vi "setWindow.vi"(8 "error in (no error)":errorcluster, 10 "Window Number (0...15)":i32, 11 "Stimulus in":refnum<class "Stimulus.lvclass">) -> (0 "error out":errorcluster, 3 "Stimulus out":refnum<class "Stimulus.lvclass">)   [LabVIEW 2013, in "Stimulus.lvclass"]
uses:
  Stimulus.lvclass
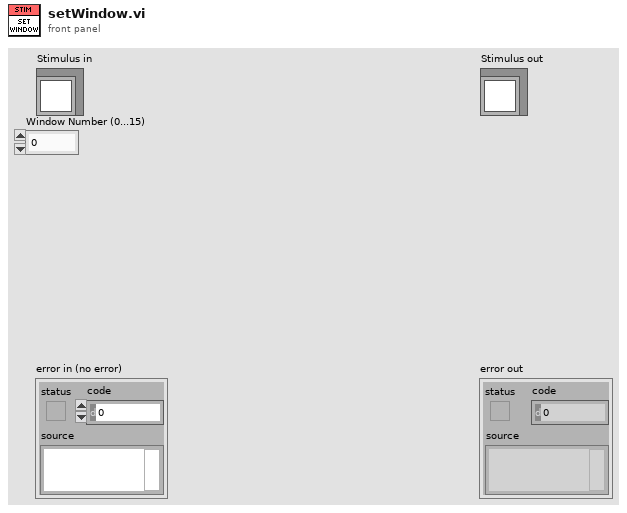
[diagram p1: front panel]
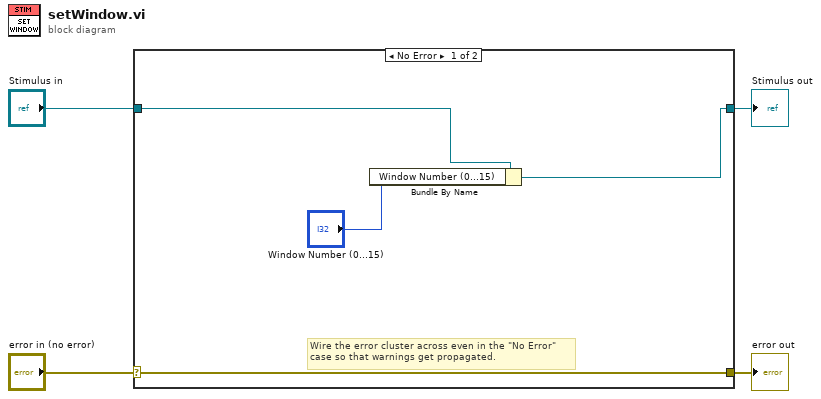
[diagram p0: block diagram]
diagram:
  n1 = case shown="No Error" "error in (no error)" {
    selector: "error in (no error)" -> [w8 w10]
    tunnel: [w8 w10] -> w3
    tunnel: [w6 w9] -> w1
    tunnel: "Stimulus in" -> [w7 w9]
    frame No Error {
      # "Wire the error cluster across even in the \"No Error\"\ncase so that warnings get propagated."
      n2 = Bundle By Name(cluster=w7, "Window Number (0...15)"="Window Number (0...15)") -> (w6:refnum<class "Stimulus.lvclass">)
    }
    frame Error {
    }
  }
  "error out" <- w3
  "Stimulus out" <- w1
